vi "close.vi"(8 "error in (no error)":errorcluster) -> (0 "error out":errorcluster)   [LabVIEW 2012]
uses:
  <instrlib>/Agilent E4981/Agilent E4981.lvlib
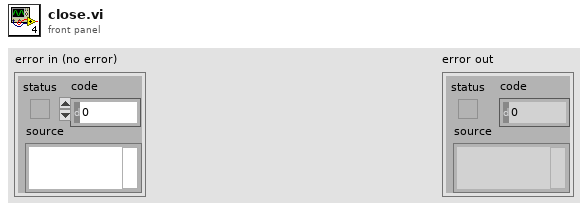
[diagram p1: front panel]
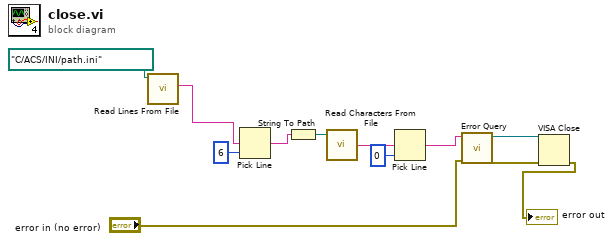
[diagram p0: block diagram]
diagram:
  n1 = call <vilib>:"Read Lines From File.vi"("file path (dialog if empty)"=path "C:/ACS/INI/path.ini") -> ("line string"=w8:string)  [unwired: 5 in, 3 out]
  n2 = Pick Line(multi-line string=w8, line index=6) -> (output string=w10:string)  [unwired: 1 in]
  n3 = String To Path(string=w10) -> (path=w9:path)
  n4 = call <vilib>:"Read Characters From File.vi"("file path (dialog if empty)"=w9) -> ("character string"=w7:string)  [unwired: 5 in, 3 out]
  n5 = Pick Line(multi-line string=w7, line index=0) -> (output string=w5:string)  [unwired: 1 in]
  n6 = call <instrlib>:"Error Query.vi"("error in (no error)"="error in (no error)", "VISA resource name"=w5) -> ("error out"=w3:errorcluster, "VISA resource name out"=w4:refnum<visa-resource-name>)  [unwired: 6 in, 2 out]
  n7 = VISA Close(VISA resource name=w4, error in (no error)=w3) -> (error out=→"error out":errorcluster)
